vi "readFromXML.vi"(8 "error in (no error)":errorcluster, 10 "XML in":string, 11 "MccEnable in":refnum<class "MccEnable.lvclass">) -> (0 "error out":errorcluster, 3 "MccEnable out":refnum<class "MccEnable.lvclass">)   [LabVIEW 2022 SP3, in "TCSDataDefinitions.lvlib" / "TCSMountControlCommand.lvlib" / "CommandsForAllAxes.lvlib" / "MccEnable.lvclass"]
uses:
  MccEnable.lvclass
  CommandsForAllAxes.lvclass
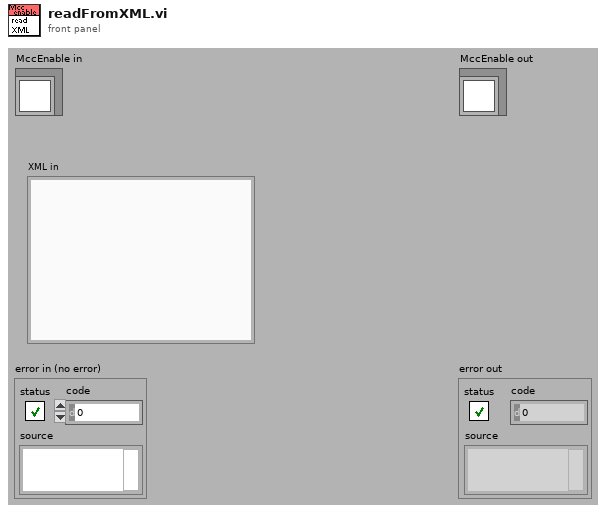
[diagram p1: front panel]
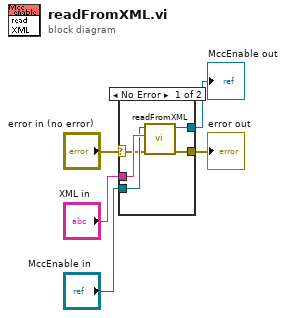
[diagram p0: block diagram]
diagram:
  n1 = case shown="No Error" "error in (no error)" {
    selector: "error in (no error)" -> [w6 w12]
    tunnel: [w10 w12] -> w5
    tunnel: [w9 w11] -> w4
    tunnel: "XML in" -> [w8 _]
    tunnel: "MccEnable in" -> [w7 w11]
    frame No Error {
      n2 = call-parent "readFromXML.vi"("error in (no error)"=w6, "XML in"=w8, "CommandsForAllAxes in"=w7) -> ("error out"=w10:errorcluster, "CommandsForAllAxes out"=w9:refnum<class "MccEnable.lvclass">)  [unwired: 7 out]
    }
    frame Error {
    }
  }
  "error out" <- w5
  "MccEnable out" <- w4
